vi "JSONRPC-GetCamerasInfo.vi"(11 "expId":string) -> (3 "Output":string[](array[string]))   [LabVIEW 2015]
uses:
  Configuration/Global_Configurations.vi
panel:
  # "GetCamerasInfo"
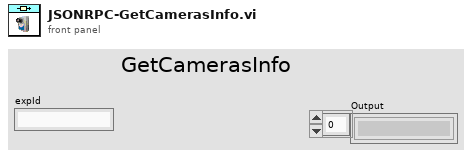
[diagram p1: front panel]
types:
  T1 = cluster{"Path":path, "Name":string, "Authors":string, "Keywords":string, "Description":string, "Cameras":cluster{"Base URL":string, "Path":string, "Name":string}[]}[]
  T2 = cluster{"Base URL":string, "Path":string, "Name":string}[]
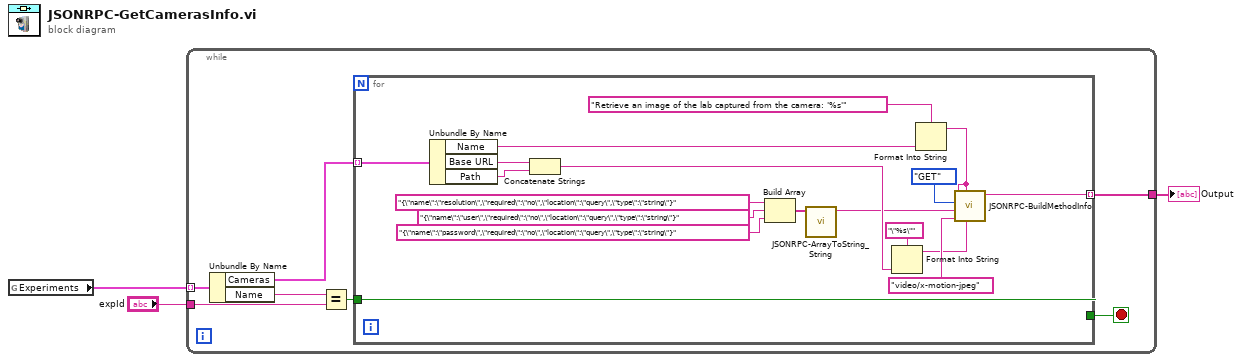
[diagram p0: block diagram]
diagram:
  n1 = global read "Global_Configurations.vi" "Experiments"() -> (w2:T1)
  n2 = while {
    tunnel: w2 -> [w10] mode=indexing
    tunnel: "expId" -> [w9]
    tunnel: [w5] -> w1
    stop <- w7 stop-if-true
    n3 = Unbundle By Name(w10) -> ("Cameras"=w4:T2, "Name"=w8:string)
    n4 = Equal?(x=w8, y=w9) -> (x = y?=w6:bool)
    n5 = for {
      tunnel: [w28] -> w7
      tunnel: w6 -> [w28]
      tunnel: [w21] -> w5 mode=indexing
      tunnel: w4 -> [w19] mode=indexing
      n6 = Unbundle By Name(w19) -> ("Name"=w17:string, "Base URL"=w16:string, "Path"=w15:string)
      n7 = Concatenate Strings(w16, w15) -> (w14:string)
      n8 = Build Array("{\"name\":\"resolution\",\"required\":\"no\",\"location\":\"query\",\"type\":\"string\"}" ("Params"), "{\"name\":\"user\",\"required\":\"no\",\"location\":\"query\",\"type\":\"string\"}" ("Params"), "{\"name\":\"password\",\"required\":\"no\",\"location\":\"query\",\"type\":\"string\"}" ("Params")) -> (w23:string[])
      n9 = call "JSONRPC-ArrayToString_String.vi"("Array"=w23) -> ("Output"=w13:string)  [unwired: 10 in]
      n10 = Format Into String(format string="\"%s\"", w14) -> (resulting string=w12:string)  [unwired: 2 in, 1 out]
      n11 = Format Into String(format string="Retrieve an image of the lab captured from the camera: '%s'" ("Description"), w17) -> (resulting string=w11:string)  [unwired: 2 in, 1 out]
      n12 = call "JSONRPC-BuildMethodInfo.vi"("Example"=w12, "Description"=w11, "Returns"="video/x-motion-jpeg", "Params"=w13, "Method"=enum16{"SSE", "GET", "POST"}."GET", "url"=w11) -> ("String"=w21:string)  [unwired: 5 in]
    }
  }
  "Output" <- w1
